vi "MGCC_FntStaMach_Initial_additional_functions.vi"   [LabVIEW 2016]
doc: "This VI is designed to give the enable buttons for all the subfuctions according to project."
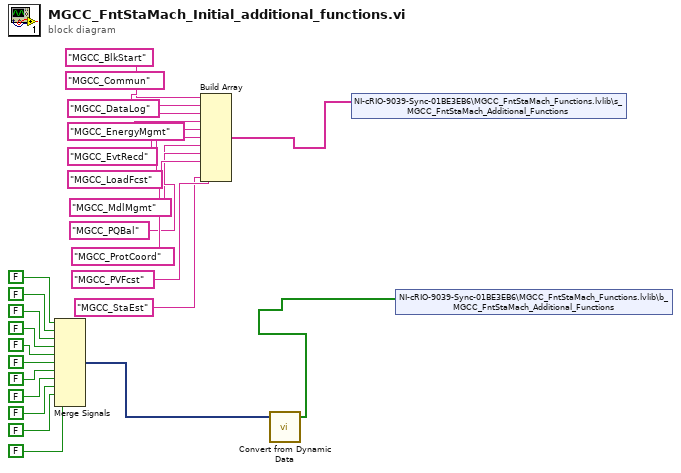
[diagram p0: block diagram]
diagram:
  n1 = Merge Signals(FALSE ("State3"), FALSE ("State3"), FALSE ("State3"), FALSE ("State3"), FALSE ("State3"), FALSE ("State3"), FALSE ("State3"), FALSE ("State3"), FALSE ("State3"), FALSE ("State3"), FALSE ("State3")) -> (w15:dynamicdata)
  n2 = Build Array("MGCC_BlkStart", "MGCC_Commun", "MGCC_DataLog", "MGCC_EnergyMgmt", "MGCC_EvtRecd", "MGCC_LoadFcst", "MGCC_MdlMgmt", "MGCC_PQBal", "MGCC_ProtCoord", "MGCC_PVFcst", "MGCC_StaEst") -> (w3:string[])
  n3 = call "Convert from Dynamic Data"("Dynamic Data Type"=w15) -> ("Array"=w1:bool[])  [unwired: 3 in]
  n4 = shared-variable "NI-cRIO-9039-Sync-01BE3EB6\\MGCC_FntStaMach_Functions.lvlib\\s_MGCC_FntStaMach_Additional_Functions"(w3) -> ()  [unwired: 1 in, 1 out]
  n5 = shared-variable "NI-cRIO-9039-Sync-01BE3EB6\\MGCC_FntStaMach_Functions.lvlib\\b_MGCC_FntStaMach_Additional_Functions"(w1) -> ()  [unwired: 1 in, 1 out]
